vi "Day 3.vi"() -> ()   [LabVIEW 2023]
panel:
  out "sum":dbl
  out "Array 2":dbl[](array[numeric])
  out "Array":string[](array[string])
  out "array":string[](array[string])
  in  "input":string="vJrwpWtwJgWrhcsFMMfFFhFp\njqHRNqRjqzjGDLGLrsFMfFZSrLrFZsSL\nPmmdzqPrVvPwwTWBwg\nwMqvLMZHhHMvwLHjbvcjnnSBnvTQFn\nttgJtRGJQctTZtZT\nCrZsJsPPZsGzwwsLwLmpwMDw"
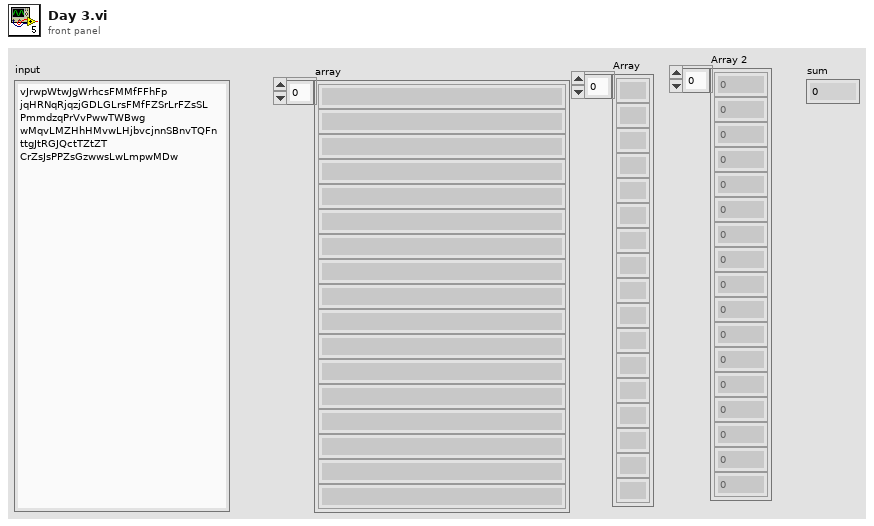
[diagram p1: front panel]
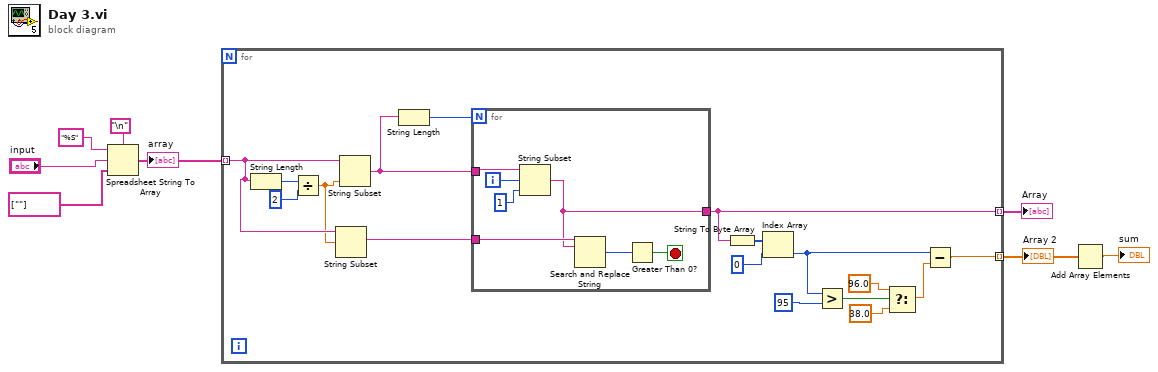
[diagram p0: block diagram]
diagram:
  n1 = Spreadsheet String To Array(delimiter (Tab)="\n", format string="%S", spreadsheet string="input", array type (2D Dbl)=string[] [""]) -> (array=w4:string[])
  "array" <- w4
  n2 = for {
    tunnel: w4 -> [w23] mode=indexing
    tunnel: [w18] -> w3 mode=indexing
    tunnel: [w10] -> w2 mode=indexing
    n3 = String Length(string=w23) -> (length=w25:i32)
    n4 = Divide(x=w25, y=2) -> (x/y=w22:dbl)
    n5 = String Subset(string=w23, offset (0)=w22) -> (substring=w19:string)  [unwired: 1 in]
    n6 = String Subset(string=w23, length (rest)=w22) -> (substring=w20:string)  [unwired: 1 in]
    n7 = String Length(string=w20) -> (length=w21:i32)
    n8 = for {
      N: w21 -> [_]
      tunnel: w20 -> [w31]
      tunnel: w19 -> [w32]
      tunnel: [w26] -> w18
      i -> [w30]
      stop <- w27 stop-if-true
      n9 = String Subset(string=w31, offset (0)=w30, length (rest)=1 ("length (rest)")) -> (substring=w26:string)
      n10 = Search and Replace String(input string=w32, search string=w26) -> (number of replacements=w28:i32)  [unwired: 6 in, 3 out]
      n11 = Greater Than 0?(x=w28) -> (x > 0?=w27:bool)
    }
    n12 = String To Byte Array(string=w18) -> (unsigned byte array=w11:u8[])
    n13 = Index Array(array=w11, index=0) -> (element=w9:u8)
    n14 = Greater?(x=w9, y=u8 95) -> (0:w15:bool)
    n15 = Select(t=96.0, s=w15, f=38.0) -> (s? t:f=w12:dbl)
    n16 = Subtract(x=w9, y=w12) -> (x-y=w10:dbl)
  }
  "Array" <- w3
  "Array 2" <- w2
  n17 = Add Array Elements(numeric array=w2) -> (sum=→"sum":dbl)
